vi "Roughness Averager Watershed Compute.vi"(8 "error in (no error)":errorcluster, 9 "Connectivity 4/8 (4)":bool=TRUE, 10 "Grayscale Image":T1, 11 "Roughness Averager in":refnum<class "Roughness Averager.lvclass">) -> (0 "error out":errorcluster, 3 "Roughness Averager out":refnum<class "Roughness Averager.lvclass">)   [LabVIEW 2018, in "Roughness Averager.lvclass"]
uses:
  Roughness Averager.lvclass
  <vilib>/vision/Image Controls.llb/IMAQ Image.ctl
  Roughness Averager.lvclass/Roughness Averager.ctl
panel:
  in  "Watershed Image Name":string="untitled"
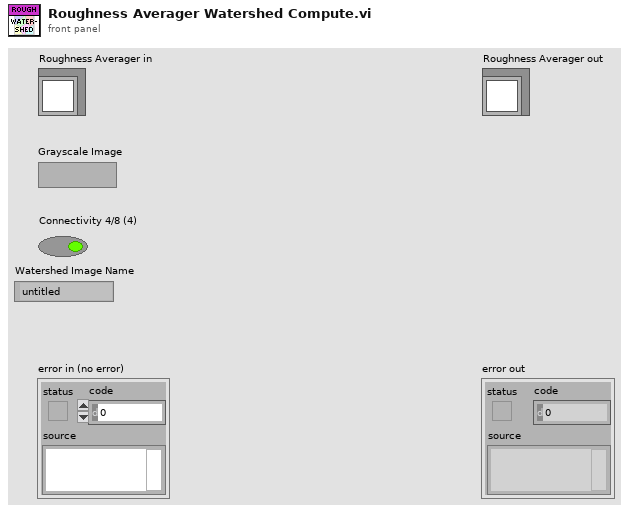
[diagram p1: front panel]
types:
  T1 = typedef "IMAQ Image.ctl" = refnum<image>
  T2 = cluster{"Area":dbl, "Number of Holes":dbl, "Bounding Rect":cluster{"Left":dbl, "Top":dbl, "Right":dbl, "Bottom":dbl}, "Center of Mass":cluster{"X":dbl, "Y":dbl}, "Orientation":dbl, "Dimensions":cluster{"Width":dbl, "Height":dbl}}[]
  T3 = cluster{"Image Dst Out":T1, "Number of Zones":i32, "Particle Reports (Pixels)":cluster{"Area":dbl, "Number of Holes":dbl, "Bounding Rect":cluster{"Left":dbl, "Top":dbl, "Right":dbl, "Bottom":dbl}, "Center of Mass":cluster{"X":dbl, "Y":dbl}, "Orientation":dbl, "Dimensions":cluster{"Width":dbl, "Height":dbl}}[]}
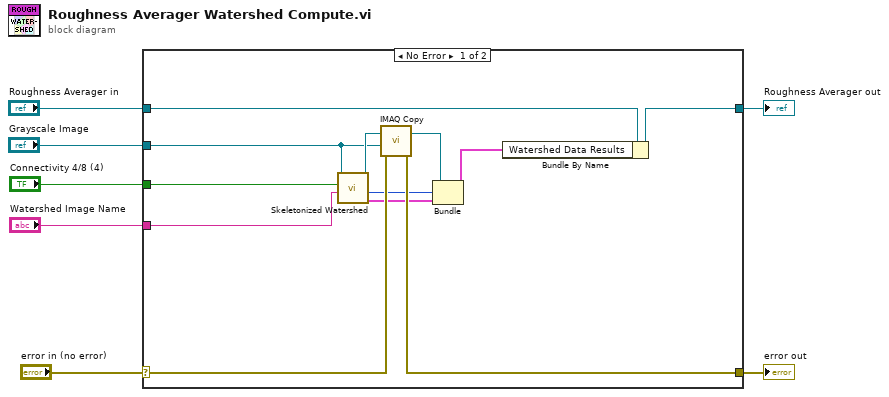
[diagram p0: block diagram]
diagram:
  n1 = case shown="No Error" "error in (no error)" {
    selector: "error in (no error)" -> [w15 w21]
    tunnel: [w14 w21] -> w6
    tunnel: [w8 w20] -> w4
    tunnel: "Roughness Averager in" -> [w10 w20]
    tunnel: "Grayscale Image" -> [w16 _]
    tunnel: "Connectivity 4/8 (4)" -> [w19 _]
    tunnel: "Watershed Image Name" -> [w18 _]
    frame No Error {
      n2 = call "Skeletonized Watershed.vi"("Image Name"=w18, "Connectivity 4/8 (4)"=w19, "Grayscale Image"=w16) -> ("Particle Reports (Pixels)"=w11:T2, "Number of Zones"=w12:i32, "Image Out"=w17:T1)  [unwired: 6 in]
      n3 = call "IMAQ Copy"("error in (no error)"=w15, "Image Dst"=w16, "Image Src"=w17) -> ("error out"=w14:errorcluster, "Image Dst Out"=w13:T1)  [unwired: 3 in]
      n4 = Bundle("Image Dst Out"=w13, "Number of Zones"=w12, "Particle Reports (Pixels)"=w11) -> (w9:T3)  [unwired: 1 in]
      n5 = Bundle By Name(cluster=w10, "Watershed Data Results"=w9) -> (w8:refnum<class "Roughness Averager.lvclass">)
    }
    frame Error {
    }
  }
  "error out" <- w6
  "Roughness Averager out" <- w4
